vi "Get Array Element TDEnum.vi"(8 "错误输入":errorcluster, 11 "Array":variant) -> (0 "错误输出":errorcluster, 3 "Type Code":T1 format="%02x")   [LabVIEW 2012, in "TD Tools.lvlib"]
uses:
  TD Tools.lvlib
  Custom Type/Type Descriptor Enumeration.ctl
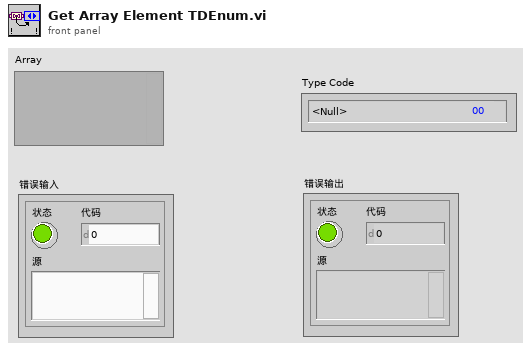
[diagram p1: front panel]
types:
  T1 = typedef "TD Tools.lvlib/Type Descriptor Enumeration.ctl" = enum16{"<Null>", "I8", "I16", "I32", "I64", "U8", "U16", "U32", "U64", "SGL", "DBL", "EXT", "CSG", "CDB", "CXT", "0x0F", "0x10", "0x11", "0x12", "0x13", "0x14", "Enum U8", "Enum U16", "Enum U32", "Enum U64", "SGL PQ", "DBL PQ", "EXT PQ", "CSG PQ", "CDB PQ", "CXT PQ", "0x1F", "0x20", "Boolean", "0x22", "0x23", "0x24", "0x25", "0x26", "0x27", "0x28", "0x29", "0x2A", "0x2B", "0x2C", "0x2D", "0x2E", "0x2F", "String", "0x31", "Path", "Pict", "0x34", "0x35", "0x36", "DAQ", "0x38", "0x39", "0x3A", "0x3B", "0x3C", "0x3D", "0x3E", "0x3F", "Array", "0x41", "0x42", "0x43", "0x44", "0x45", "0x46", "0x47", "0x48", "0x49", "0x4A", "0x4B", "0x4C", "0x4D", "0x4E", "0x4F", "Cluster", "0x51", "0x52", "Variant", "Waveform", "0x55", "0x56", "0x57", "0x58", "0x59", "0x5A", "0x5B", "0x5C", "0x5D", "0x5E", "0x5F", "0x60", "0x61", "0x62", "0x63", "0x64", "0x65", "0x66", "0x67", "0x68", "0x69", "0x6A", "0x6B", "0x6C", "0x6D", "0x6E", "0x6F", "Refnum"}
  T2 = typedef "TD Tools.lvlib/Type Descriptor.ctl" = u16[]
  T3 = typedef "TD Tools.lvlib/Type Descriptor Header.ctl" = cluster{"length":u16, "private":u8, "type":T1, "# elements":u16}
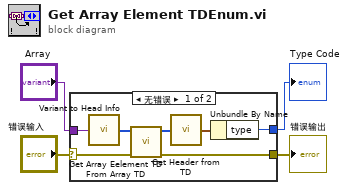
[diagram p0: block diagram]
diagram:
  n1 = case shown="无错误" "错误输入" {
    selector: "错误输入" -> [w6 w12]
    tunnel: "Array" -> [w11 _]
    tunnel: [w7 _] -> w3
    tunnel: [w5 w12] -> w1
    frame No Error {
      n2 = call "Variant to Head Info.vi"("Variant"=w11) -> ("Type Descriptor"=w10:T2)  [unwired: 2 in, 2 out]
      n3 = call "Get Array Eelement TD From Array TD.vi"("错误输入"=w6, "Array Type Descriptor"=w10) -> ("错误输出"=w5:errorcluster, "Element Type Descriptor"=w9:T2)  [unwired: 8 in]
      n4 = call "Get Header from TD.vi"("Type Desciptor"=w9) -> ("Type Descriptor Header"=w8:T3)
      n5 = Unbundle By Name(w8) -> ("type"=w7:T1)
    }
    frame Error {
    }
  }
  "Type Code" <- w3
  "错误输出" <- w1
